vi "GC Helium - Step 5.vi"(7 "Step":i32, 8 "error in":errorcluster, 9 "Test Results In":T8, 10 "Gas":T1, 11 "GC Configuration":T2) -> (0 "error out":errorcluster, 1 "Test Results Out":T8, 2 "Gas Out":T1 caption="Gas", 3 "GC Configuration Out":T2)   [LabVIEW 2015]
uses:
  Controls/Test Information.ctl
  Controls/Vacuum Test.ctl
  Controls/Test Timing.ctl
  Controls/Vaccum Thresholds.ctl
  Controls/Helium Test.ctl
  Controls/Helium Thresholds.ctl
  CAN Communication/Gas/Typedefs/Session Handle.ctl
  CAN Communication/Gas/Gas.lvclass
  Controls/Test Results.ctl
  Controls/Step Result.ctl
  CAN Communication/Gas/Typedefs/Valves.ctl
  SubVIs/Timing/Timing.lvlib
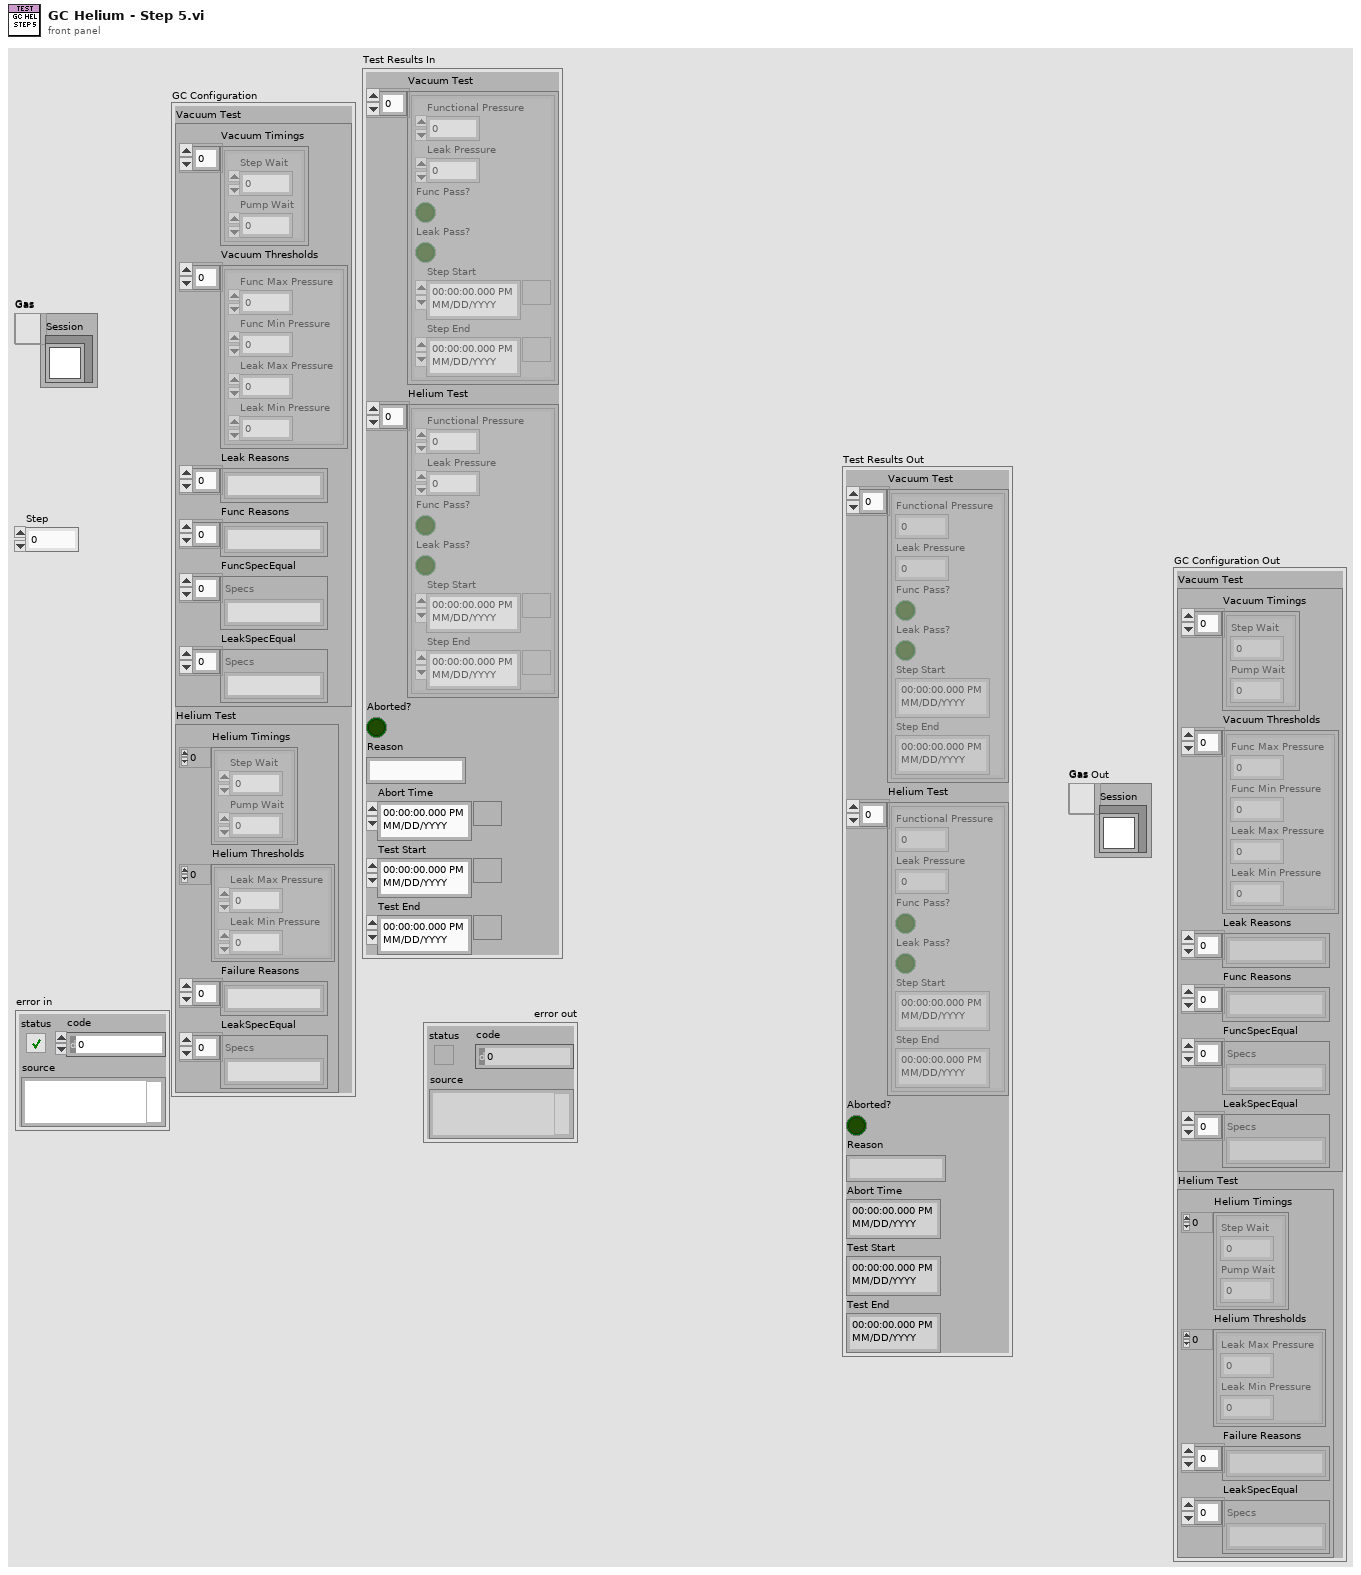
[diagram p1: front panel]
types:
  T1 = typedef "Gas.lvclass/Session Handle.ctl" = refnum<data-value>
  T2 = typedef "Test Information.ctl" = cluster{"Vacuum Test":T3, "Helium Test":T6}
  T3 = typedef "Vacuum Test.ctl" = cluster{"Vacuum Timings":T4[], "Vacuum Thresholds":T5[], "Leak Reasons":string[], "Func Reasons":string[], "FuncSpecEqual":string[], "LeakSpecEqual":string[]}
  T4 = typedef "Test Timing.ctl" = cluster{"Step Wait":dbl, "Pump Wait":dbl}
  T5 = typedef "Vaccum Thresholds.ctl" = cluster{"Func Max Pressure":dbl, "Func Min Pressure":dbl, "Leak Max Pressure":dbl, "Leak Min Pressure":dbl}
  T6 = typedef "Helium Test.ctl" = cluster{"Helium Timings":T4[], "Helium Thresholds":T7[], "Failure Reasons":string[], "LeakSpecEqual":string[]}
  T7 = typedef "Helium Thresholds.ctl" = cluster{"Leak Max Pressure":dbl, "Leak Min Pressure":dbl}
  T8 = typedef "Test Results.ctl" = cluster{"Vacuum Test":T9[], "Helium Test":T9[], "Aborted?":bool, "Reason":string, "Abort Time":timestamp, "Test Start":timestamp, "Test End":timestamp}
  T9 = typedef "Step Result.ctl" = cluster{"Functional Pressure":dbl, "Leak Pressure":dbl, "Func Pass?":bool, "Leak Pass?":bool, "Step Start":timestamp, "Step End":timestamp}
  T10 = typedef "Gas.lvclass/Valves.ctl" = u16
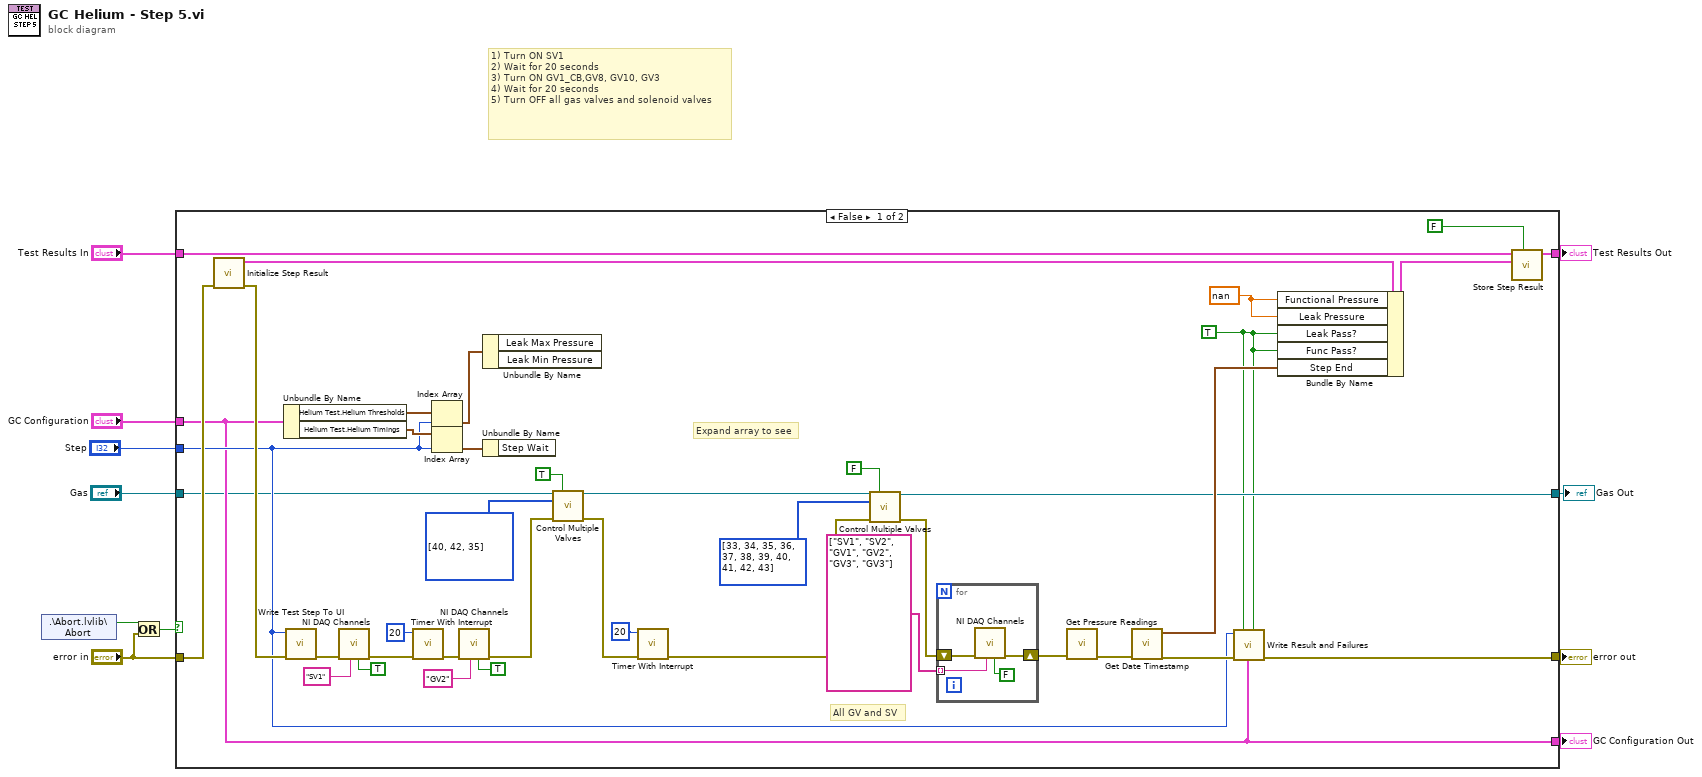
[diagram p0: block diagram]
diagram:
  # "1) Turn ON SV1\n2) Wait for 20 seconds\n3) Turn ON GV1_CB,GV8, GV10, GV3\n4) Wait for 20 seconds\n5) Turn OFF all gas valves and solenoid valves"
  n1 = shared-variable ".\\Abort.lvlib\\Abort"() -> (w10:bool)  [unwired: 1 in, 1 out]
  n2 = Or(x=w10, y="error in") -> (x .or. y?=w9:bool)
  n3 = case shown="False" w9 {
    tunnel: "error in" -> [w52 w59]
    tunnel: "Test Results In" -> [w49 w60]
    tunnel: [w50 w60] -> w7
    tunnel: [w39 w59] -> w6
    tunnel: "GC Configuration" -> [w37 w58]
    tunnel: "Step" -> [w38 _]
    tunnel: [w37 w58] -> w3
    tunnel: [w30 w57] -> w1
    tunnel: "Gas" -> [w34 w57]
    frame False {
      w24 = T10[] [33, 34, 35, 36, 37, 38, 39, 40, 41, 42, 43] items=["GV1"=33, "GV2"=34, "GV3"=35, "GV4"=36, "GV5"=37, "GV6"=38, "GV7"=39, "GV8"=40, "GV9"=41, "GV10"=42, "GV11"=43, "LV3"=51, "LV4"=52] ("Valves")
      w28 = T10[] [40, 42, 35] items=["GV1"=33, "GV2"=34, "GV3"=35, "GV4"=36, "GV5"=37, "GV6"=38, "GV7"=39, "GV8"=40, "GV9"=41, "GV10"=42, "GV11"=43, "LV3"=51, "LV4"=52] ("Valves")
      w26 = TRUE ("Func Pass?")
      w15 = nan ("Functional Pressure")
      # "Expand array to see"
      # "All GV and SV"
      n4 = call "Initialize Step Result.vi"("error in (no error)"=w52) -> ("error out"=w51:errorcluster, "New Step Result"=w48:T9)  [unwired: 8 in, 1 out]
      n5 = Unbundle By Name(w37) -> ("Helium Test.Helium Thresholds"=w45:T7[], "Helium Test.Helium Timings"=w44:T4[])
      n6 = call "Write Test Step To UI.vi"("error in (no error)"=w51, "Step"=w38) -> ("error out"=w22:errorcluster)  [unwired: 9 in]
      n7 = call "NI DAQ Channels.vi"("Control"=TRUE ("State"), "Channel"="SV1", "error in (no error)"=w22) -> ("error out"=w21:errorcluster)  [unwired: 7 in, 1 out]
      n8 = call "Timer With Interrupt.vi"("error in (no error)"=w21, "Wait (s)"=20) -> ("error out"=w19:errorcluster)  [unwired: 7 in, 2 out]
      n9 = Index Array(array=w45, index=w38) -> (element=w41:T7)
      n10 = Index Array(array=w44, index=w38) -> (element=w43:T4)
      n11 = call "NI DAQ Channels.vi"("Control"=TRUE ("State"), "Channel"="GV2", "error in (no error)"=w19) -> ("error out"=w18:errorcluster)  [unwired: 7 in, 1 out]
      n12 = Unbundle By Name(w41) -> ()  [unwired: 2 out]
      n13 = Unbundle By Name(w43) -> ()  [unwired: 1 out]
      n14 = call "Control Multiple Valves.vi"("Session Handle in"=w34, "Energize?"=TRUE, "Valves"=w28, "error in (no error)"=w18) -> ("Session Handle out"=w31:T1, "error out"=w32:errorcluster)  [unwired: 8 in, 2 out]
      n15 = call "Timer With Interrupt.vi"("error in (no error)"=w32, "Wait (s)"=20) -> ("error out"=w25:errorcluster)  [unwired: 7 in, 2 out]
      n16 = call "Control Multiple Valves.vi"("Session Handle in"=w31, "Energize?"=FALSE, "Valves"=w24, "error in (no error)"=w25) -> ("Session Handle out"=w30:T1, "error out"=w27:errorcluster)  [unwired: 8 in, 2 out]
      n17 = for {
        shift-right: [w53] -> w17
        shift-left: w27 -> [w54]
        tunnel: string[] ["SV1", "SV2", "GV1", "GV2", "GV3", "GV3"] -> [w56] mode=indexing
        n18 = call "NI DAQ Channels.vi"("Control"=FALSE ("data"), "Channel"=w56, "error in (no error)"=w54) -> ("error out"=w53:errorcluster)  [unwired: 7 in, 1 out]
      }
      n19 = call "Get Pressure Readings.vi"("error in (no error)"=w17) -> ("error out"=w16:errorcluster)  [unwired: 6 in, 4 out]
      n20 = call "Get Date Timestamp.vi"("error in (no error)"=w16) -> ("error out"=w40:errorcluster, "current time"=w46:timestamp)  [unwired: 9 in]
      n21 = call "Write Result and Failures.vi"("Leak"=w26, "GC Configuration"=w37, "Func"=w26, "error in (no error)"=w40, "Step"=w38) -> ("error out"=w39:errorcluster)  [unwired: 6 in]
      n22 = Bundle By Name(cluster=w48, "Functional Pressure"=w15, "Leak Pressure"=w15, "Leak Pass?"=w26, "Func Pass?"=w26, "Step End"=w46) -> (w47:T9)
      n23 = call "Store Step Result.vi"("Vacuum?"=FALSE, "Step Result"=w47, "Test Results In"=w49) -> ("Test Results Out"=w50:T8)  [unwired: 8 in]
    }
    frame True {
    }
  }
  "error out" <- w6
  "Test Results Out" <- w7
  "GC Configuration Out" <- w3
  "Gas Out" <- w1
